vi "CAN input.vi"(8 "error in (no error)":errorcluster, 11 "CANopen":refnum<class "CANopen.lvclass">) -> (0 "error out":errorcluster, 2 "Input image":u8[](array[numeric]), 3 "CANopen dup":refnum<class "CANopen.lvclass">)   [LabVIEW 2017, in "canopen.lvlib" / "CANopen.lvclass"]
doc: "Returns a copy of the internally owned input image. This does not trigger any action: it merely returns the *actual* status of the inputs."
uses:
  CANopen.lvclass
  CANopen.lvclass/CANopen.ctl
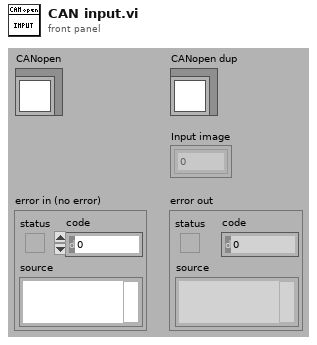
[diagram p1: front panel]
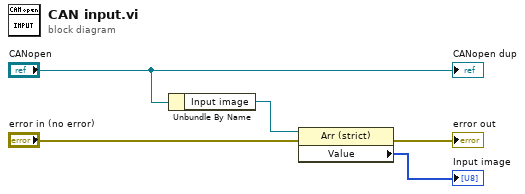
[diagram p0: block diagram]
diagram:
  n1 = Unbundle By Name("CANopen") -> ("Input image"=w2:refnum<vi>)
  n2 = property class="Arr (strict)"(reference=w2, error in="error in (no error)") -> (error out=→"error out":errorcluster, "Value"=→"Input image":u8[])  [unwired: 1 out]
  "CANopen dup" <- "CANopen"
